vi "scan-value-from-msg.vi"(8 "error in (no error)":errorcluster, 10 "msg length":u32, 11 "read buffer in":string) -> (0 "error out":errorcluster, 2 "Raw Data":dbl, 3 "read buffer out":string)   [LabVIEW 2024]
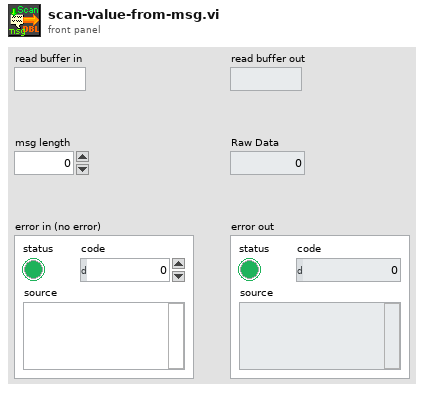
[diagram p1: front panel]
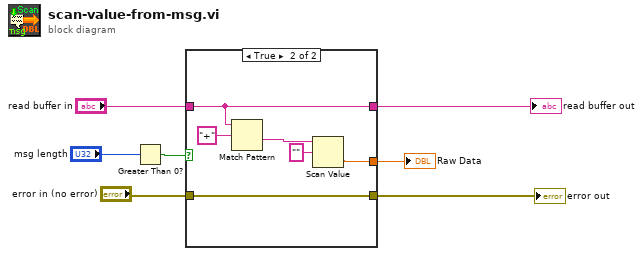
[diagram p0: block diagram]
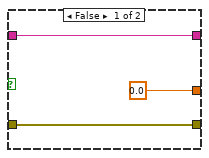
[diagram p2: hidden frame]
diagram:
  n1 = Greater Than 0?(x="msg length") -> (x > 0?=w2:bool)
  n2 = case shown="True" w2 {
    tunnel: "read buffer in" -> [w10 w15]
    tunnel: "error in (no error)" -> [w9 w16]
    tunnel: [w9 w16] -> w4
    tunnel: [w10 w15] -> w6
    tunnel: [0.0 w12] -> w7
    frame False {
    }
    frame True {
      n3 = Match Pattern(string=w15, regular expression="+") -> (after substring=w13:string)  [unwired: 1 in, 3 out]
      n4 = Scan Value(string=w13, format string="") -> (value=w12:dbl)  [unwired: 1 in, 1 out]
    }
  }
  "Raw Data" <- w7
  "read buffer out" <- w6
  "error out" <- w4
